vi "fix supported types and targets.vi"(8 "error in":errorcluster, 10 "DecideProjectFeatures in":refnum<class "UserTBModuleDecideFeatures.lvclass">, 11 "User Project in":refnum<vi>) -> (0 "error out":errorcluster, 3 "User Project out":refnum<vi>)   [LabVIEW 2013, in "UserTBModuleDecideFeatures.lvclass"]
uses:
  UserTBModuleDecideFeatures.lvclass
  UserTBModuleDecideFeatures.lvclass/UserTBModuleDecideFeatures.ctl
  Read supported data types.vi
  Read supported targets.vi
  Read instances allowed.vi
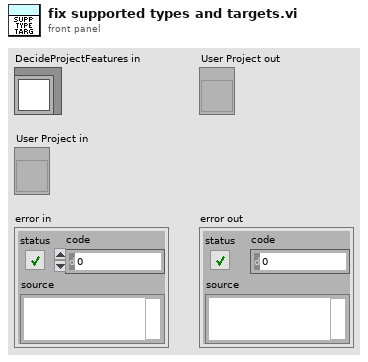
[diagram p1: front panel]
types:
  T1 = typedef "tag bus.lvlib/tag descriptor.lvclass/Data Type.ctl" = enum16{"Double", "Single", "I64", "I32", "I16", "I8", "U64", "U32", "U16", "U8", "Boolean", "String", "Array of Double", "Array of Single", "Array of I64", "Array of I32", "Array of I16", "Array of I8", "Array of U64", "Array of U32", "Array of U16", "Array of U8", "Array of Boolean", "Array of String"}
  T2 = typedef "TBM configuration.lvclass/Target Types.ctl" = enum16{"Windows", "Mac", "Linux", "Linux RT ARM", "VxWorks", "Pharlap", "Other", "Linux RT x64"}
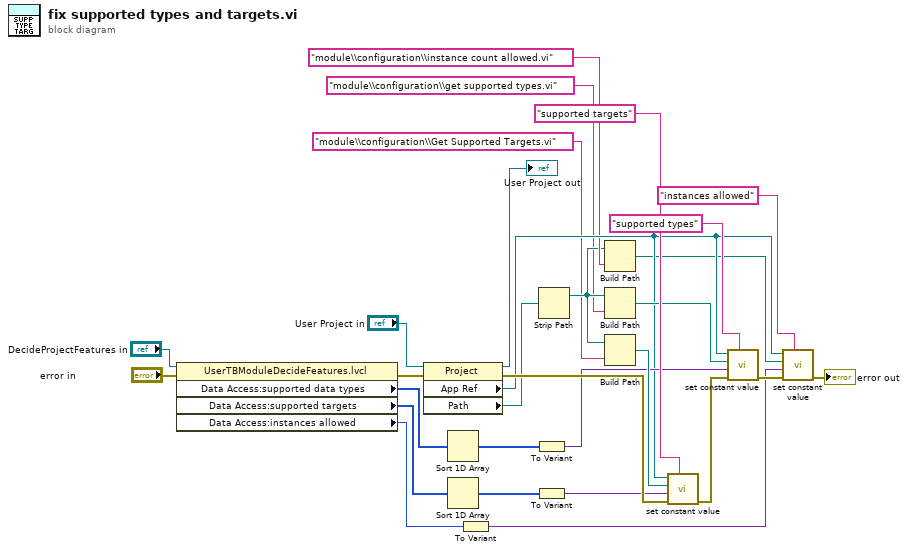
[diagram p0: block diagram]
diagram:
  n1 = property class="UserTBModuleDecideFeatures.lvcl"(reference="DecideProjectFeatures in", error in="error in") -> (error out=w23:errorcluster, "Data Access:supported data types"=w21:T1[], "Data Access:supported targets"=w22:T2[], "Data Access:instances allowed"=w9:i32)  [unwired: 1 out]
  n2 = property class="Project"(reference="User Project in", error in=w23) -> (reference out=→"User Project out":refnum<vi>, error out=w26:errorcluster, "App Ref"=w12:refnum<vi>, "Path"=w6:path)
  n3 = Sort 1D Array(array=w21) -> (sorted array=w14:T1[])
  n4 = Sort 1D Array(array=w22) -> (sorted array=w13:T2[])
  n5 = To Variant(anything=w9) -> (Variant=w8:variant)
  n6 = To Variant(anything=w14) -> (Variant=w16:variant)
  n7 = To Variant(anything=w13) -> (Variant=w19:variant)
  n8 = Strip Path(path=w6) -> (stripped path=w3:path)  [unwired: 1 out]
  n9 = Build Path(base path=w3, name or relative path="module\\configuration\\instance count allowed.vi") -> (appended path=w5:path)
  n10 = Build Path(base path=w3, name or relative path="module\\configuration\\get supported types.vi") -> (appended path=w15:path)
  n11 = Build Path(base path=w3, name or relative path="module\\configuration\\Get Supported Targets.vi") -> (appended path=w27:path)
  n12 = call "set constant value.vi"("control name"="supported targets" ("y"), "error in"=w26, "data to set"=w19, "vi path"=w27, "Application in"=w12) -> ("error out"=w17:errorcluster)  [unwired: 6 in]
  n13 = call "set constant value.vi"("control name"="supported types" ("y"), "error in"=w17, "data to set"=w16, "vi path"=w15, "Application in"=w12) -> ("error out"=w11:errorcluster)  [unwired: 6 in]
  n14 = call "set constant value.vi"("control name"="instances allowed", "error in"=w11, "data to set"=w8, "vi path"=w5, "Application in"=w12) -> ("error out"=→"error out":errorcluster)  [unwired: 6 in]
